vi "AWG Select and Initiate Script.vi"(6 "Timeout (msec)":i32=50000, 8 "error in (no error)":errorcluster, 9 "Wait for Completion":bool, 10 "script name":string, 11 "Semiconductor Module Context":T1) -> (0 "error out":errorcluster, 2 "Sessions Out":refnum<k15>[](array[refnum]), 3 "Semiconductor Module Context Out":T1)   [LabVIEW 2013]
doc: "Selects and initiates the script name selected."
uses:
  <vilib>/NI_TestStand_SemiconductorModule/NI_TestStand_Semiconductor_Module.lvlibp/PinMap/General/SemiconductorModuleContext.ctl
  <vilib>/NI_TestStand_SemiconductorModule/NI_TestStand_Semiconductor_Module.lvlibp
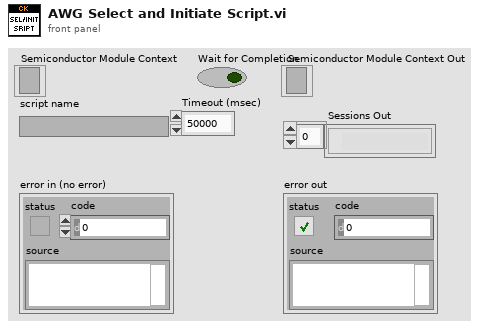
[diagram p1: front panel]
types:
  T1 = typedef "NI_TestStand_Semiconductor_Module.lvlibp/SemiconductorModuleContext.ctl" = refnum<k7>
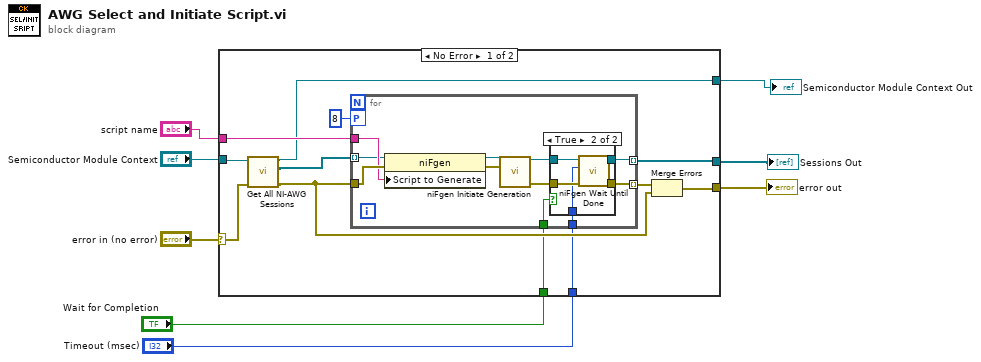
[diagram p0: block diagram]
diagram:
  n1 = case shown="No Error" "error in (no error)" {
    selector: "error in (no error)" -> [w14 w40]
    tunnel: "Semiconductor Module Context" -> [w12 w39]
    tunnel: "script name" -> [w20 _]
    tunnel: [w18 w40] -> w6
    tunnel: [w17 _] -> w4
    tunnel: "Wait for Completion" -> [w11 _]
    tunnel: "Timeout (msec)" -> [w10 _]
    tunnel: [w9 w39] -> w1
    frame No Error {
      n2 = call "Get All NI-AWG Sessions.vi"("error in (no error)"=w14, "Semiconductor Module Context"=w12) -> ("error out"=w15:errorcluster, "Instrument Sessions"=w13:refnum<k15>[], "Semiconductor Module Context Out"=w9:T1)  [unwired: 7 in]
      n3 = for {
        tunnel: w15 -> [w31]
        tunnel: w20 -> [w28]
        tunnel: [w25] -> w19 mode=indexing
        tunnel: [w26] -> w17 mode=indexing
        workers-P: 8 -> [_]
        tunnel: w13 -> [w27] mode=indexing
        tunnel: w11 -> [w22]
        tunnel: w10 -> [w21]
        n4 = property class="niFgen"(reference=w27, error in=w31, "Script to Generate"=w28) -> (reference out=w29:refnum<k15>, error out=w30:errorcluster)
        n5 = call <instrlib>:"niFgen Initiate Generation.vi"("error in (no error)"=w30, "Instrument Handle"=w29) -> ("error out"=w23:errorcluster, "Instrument Handle Out"=w24:refnum<k15>)  [unwired: 8 in]
        n6 = case shown="True" w22 {
          tunnel: [w33 w38] -> w26
          tunnel: [w32 w37] -> w25
          tunnel: w24 -> [w33 w36]
          tunnel: w23 -> [w32 w35]
          tunnel: w21 -> [_ w34]
          frame False {
          }
          frame True {
            n7 = call <instrlib>:"niFgen Wait Until Done.vi"("error in (no error)"=w35, "MaxTime (msec)"=w34, "Instrument Handle"=w36) -> ("error out"=w37:errorcluster, "Instrument Handle Out"=w38:refnum<k15>)  [unwired: 7 in]
          }
        }
      }
      n8 = Merge Errors(w19, w15) -> (w18:errorcluster)
    }
    frame Error {
    }
  }
  "error out" <- w6
  "Sessions Out" <- w4
  "Semiconductor Module Context Out" <- w1
